vi "GetNamedPosition.vi"(8 "error in (no error)":errorcluster, 10 "Name":string, 11 "XYStage":refnum<class "XYStage.lvclass">) -> (0 "error out":errorcluster, 1 "exists":bool, 2 "Position":T1, 3 "XYStage out":refnum<class "XYStage.lvclass">)   [LabVIEW 2013, in "XYStage.lvclass"]
doc: "---------------------------------------------------------------\nJKI State Machine Objects™\nhttp://jki.net/state-machine-objects/\nCopyright (C) 2005-2015, JKI <info@jki.net>\nALL RIGHTS RESERVEDJKI State Machine Objects (SMO) 1.0.0.4\nJKI - JKI\nCopyright (c) 2015, JKI"
uses:
  XYStage.lvclass
  <vilib>/JKI/JKI SMO/SMO.Dictionary/SMO.Dictionary.lvclass
  Typedefs/(real)Coords--Cluster.ctl
panel:
  # "For instructions on how to use the JKI State Machine Objects, examples and video tutorials, visit:\nhttp://jki.net/state-machine-objects/\n\nJKI State Machine Objects™\nhttp://jki.net/state-machine-objects/\nCopyright (C) 2005-2015, JKI <info@jki.net>\nALL RIGHTS RESERVED"
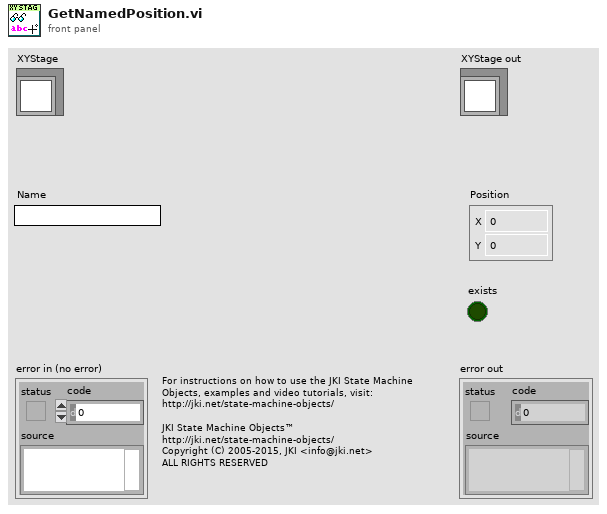
[diagram p1: front panel]
types:
  T1 = typedef "XYStage.lvclass/(real)Coords--Cluster.ctl" = cluster{"X":dbl, "Y":dbl}
  T2 = typedef "XYStage.lvclass/Dependencies--Cluster.ctl" = cluster{"Positions":refnum<class "SMO.Dictionary.Variant.lvclass">}
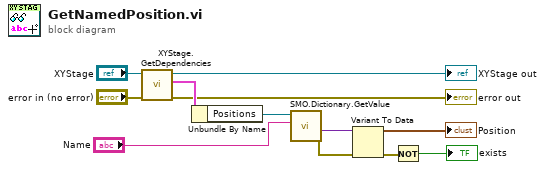
[diagram p0: block diagram]
diagram:
  n1 = call "XYStage.GetDependencies.vi"("error in (no error)"="error in (no error)", "XYStage"="XYStage") -> ("error out"=→"error out":errorcluster, "Dependencies"=w12:T2, "XYStage out"=→"XYStage out":refnum<class "XYStage.lvclass">)  [unwired: 7 in]
  n2 = Unbundle By Name(w12) -> ("Positions"=w8:refnum<class "SMO.Dictionary.Variant.lvclass">)
  n3 = call <vilib>:"SMO.Dictionary.GetValue.vi"("Key"="Name", "SMO.Dictionary"=w8) -> ("error out"=w2:errorcluster, "Value"=w6:variant)  [unwired: 5 in, 3 out]
  n4 = Variant To Data(error in=w2, Variant=w6) -> (data=→"Position":T1, error out=w4:errorcluster)  [unwired: 1 in]
  n5 = Not(x=w4) -> (.not. x?=→"exists":bool)
